vi "SingleAcquisitionClearMode.vi"() -> ()   [LabVIEW 2020]
uses:
  C:/Users/Public/Documents/Photometrics/PMQI-LabViewSamples/Examples/2018/Dependencies/PVCamNET.dll
  Dependencies/PVCamNET.dll
panel:
  in  "Exposure":u32
  out "Clear Mode":string
  in  "?":bool
  in  "?":bool
  # "SingleAcquisitionClearMode.vi\n\nDescription:\nThis sample code lets the user use single acqusition mode\nwith the user's preferred clear mode type. \n\nSteps to run:\n\n0. Before running the VI go to Window and update the Clear Mode index\n1. Click \"Run\"\n2. Enter exposure time\n3. Click \"START\"\n4. Click \"STOP\""
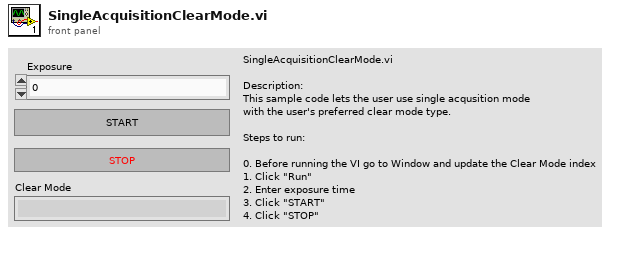
[diagram p1: front panel]
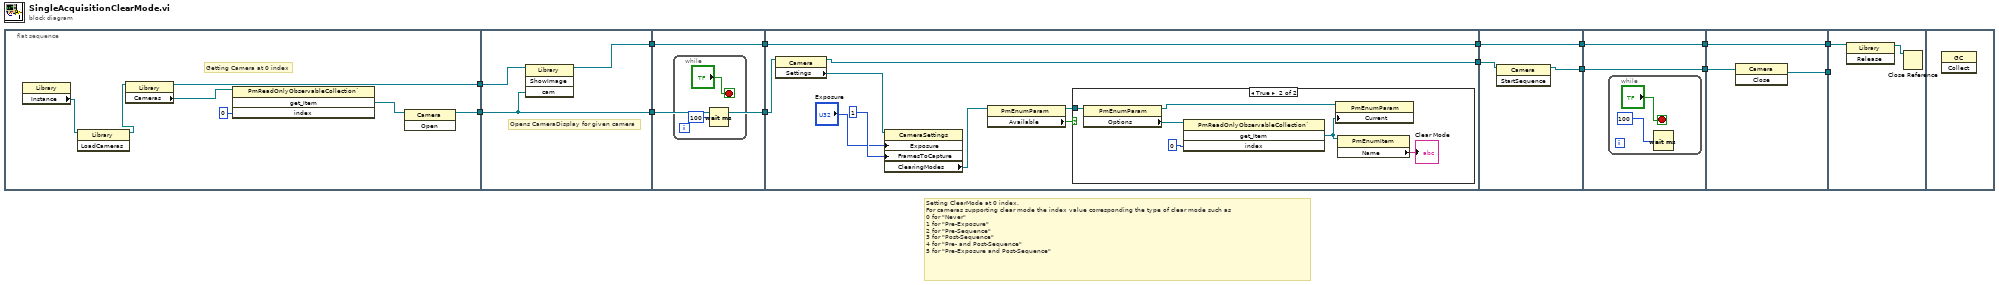
[diagram p0: block diagram]
diagram:
  # "Setting ClearMode at 0 index.\nFor cameras supporting clear mode the index value corresponding the type of clear mode such as\n0 for \"Never\"\n1 for \"Pre-Exposure\"\n2 for \"Pre-Sequence\"\n3 for \"Post-Sequence\"\n4 for \"Pre- and Post-Sequence\"\n5 for \"Pre-Exposure and Post-Sequence\""
  n1 = flat-sequence {
    tunnel: [w17] -> w14
    tunnel: [w18] -> w13
    tunnel: w14 -> [w24]
    tunnel: w13 -> [w23]
    tunnel: [w23] -> w12
    tunnel: [w22] -> w11
    tunnel: w12 -> [w26]
    tunnel: [w26] -> w9
    tunnel: w11 -> [w25]
    tunnel: [w25] -> w10
    tunnel: [w33] -> w8
    tunnel: [w37] -> w7
    tunnel: w10 -> [w37]
    tunnel: w9 -> [w34]
    tunnel: w8 -> [w45]
    tunnel: [w44] -> w6
    tunnel: [w46] -> w5
    tunnel: w7 -> [w46]
    tunnel: w6 -> [w48]
    tunnel: [w48] -> w2
    tunnel: [w47] -> w1
    tunnel: w5 -> [w47]
    tunnel: w2 -> [w53]
    tunnel: w1 -> [w51]
    tunnel: [w52] -> w4
    tunnel: [w51] -> w3
    tunnel: w4 -> [_]
    tunnel: w3 -> [w55]
    frame #0 {
      # "Getting Camera at 0 index"
      n2 = property class="Library"() -> ("Instance"=w16:refnum<k24>)  [unwired: 2 in, 2 out]
      n3 = invoke class="Library" method="LoadCameras"(reference=w16) -> (reference out=w15:refnum<k24>)  [unwired: 2 in, 2 out]
      n4 = property class="Library"(reference=w15) -> (reference out=w17:refnum<k24>, "Cameras"=w21:refnum<k24>)  [unwired: 1 in, 1 out]
      n5 = invoke class="PmReadOnlyObservableCollection`" method="get_Item"(reference=w21, "index"=0) -> ("get_Item"=w19:refnum<k24>)  [unwired: 2 in, 3 out]
      n6 = invoke class="Camera" method="Open"(reference=w19) -> (reference out=w18:refnum<k24>)  [unwired: 2 in, 2 out]
    }
    frame #1 {
      # "Opens CameraDisplay for given camera"
      n7 = invoke class="Library" method="ShowImage"(reference=w24, "cam"=w23) -> (reference out=w22:refnum<k24>)  [unwired: 2 in, 3 out]
    }
    frame #2 {
      n8 = while {
        stop <- "?" stop-if-true
        n9 = Wait (ms)(milliseconds to wait=u32 100) -> ()  [unwired: 1 out]
      }
    }
    frame #3 {
      n10 = property class="Camera"(reference=w34) -> (reference out=w33:refnum<k24>, "Settings"=w32:refnum<k24>)  [unwired: 1 in, 1 out]
      n11 = property class="CameraSettings"(reference=w32, "Exposure"="Exposure", "FramesToCapture"=u16 1) -> ("ClearingModes"=w30:refnum<k24>)  [unwired: 1 in, 2 out]
      n12 = property class="PmEnumParam"(reference=w30) -> (reference out=w35:refnum<k24>, "Available"=w36:bool)  [unwired: 1 in, 1 out]
      n13 = case shown="True" w36 {
        tunnel: w35 -> [_ w43]
        frame False {
        }
        frame True {
          n14 = property class="PmEnumParam"(reference=w43) -> (reference out=w39:refnum<k24>, "Options"=w42:refnum<k24>)  [unwired: 1 in, 1 out]
          n15 = invoke class="PmReadOnlyObservableCollection`" method="get_Item"(reference=w42, "index"=0) -> ("get_Item"=w40:refnum<k24>)  [unwired: 2 in, 3 out]
          n16 = property class="PmEnumParam"(reference=w39, "Current"=w40) -> ()  [unwired: 1 in, 2 out]
          n17 = property class="PmEnumItem"(reference=w40) -> ("Name"=→"Clear Mode":string)  [unwired: 1 in, 2 out]
        }
      }
    }
    frame #4 {
      n18 = invoke class="Camera" method="StartSequence"(reference=w45) -> (reference out=w44:refnum<k24>)  [unwired: 2 in, 2 out]
    }
    frame #5 {
      n19 = while {
        stop <- "?" stop-if-true
        n20 = Wait (ms)(milliseconds to wait=u32 100) -> ()  [unwired: 1 out]
      }
    }
    frame #6 {
      n21 = invoke class="Camera" method="Close"(reference=w53) -> (reference out=w52:refnum<k24>)  [unwired: 2 in, 2 out]
    }
    frame #7 {
      n22 = invoke class="Library" method="Release"(reference=w55) -> (reference out=w54:refnum<k24>)  [unwired: 2 in, 2 out]
      n23 = Close Reference(reference=w54) -> ()  [unwired: 1 in, 1 out]
    }
    frame #8 {
      n24 = invoke class="GC" method="Collect"() -> ()  [unwired: 3 in, 3 out]
    }
  }
